vi "Get Strings from Ref (Ryan Porter's conflicted copy 2015-04-14).vi"(8 "error in (no error)":errorcluster, 9 "Label Prefix":string, 10 "GObj Refnum in":refnum<vi>, 11 "ArrayConstant in":refnum<class "ArrayControl.lvclass">) -> (0 "error out":errorcluster, 1 "Valid?":bool, 2 "GObj Refnum out":refnum<vi>, 3 "ArrayConstant out":refnum<class "ArrayControl.lvclass">, 4 "GObj Name":string)   [LabVIEW 2013, in "SET Project Data.lvlib" / "ArrayControl.lvclass"]
uses:
  ArrayControl.lvclass
  GObject/GObject.lvclass
  SET Project Data.lvlib
  Control/Control.lvclass
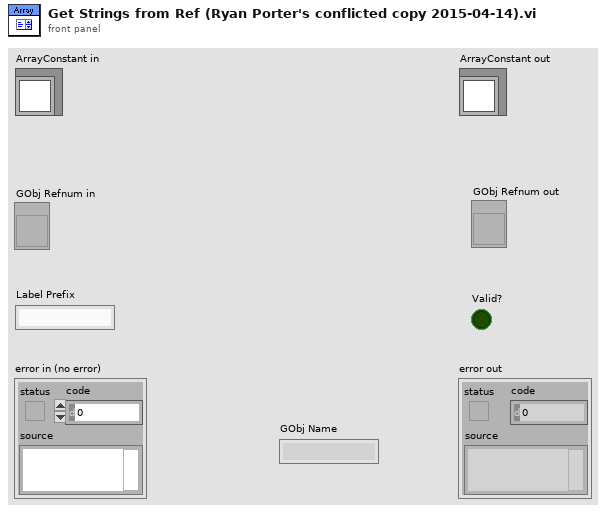
[diagram p1: front panel]
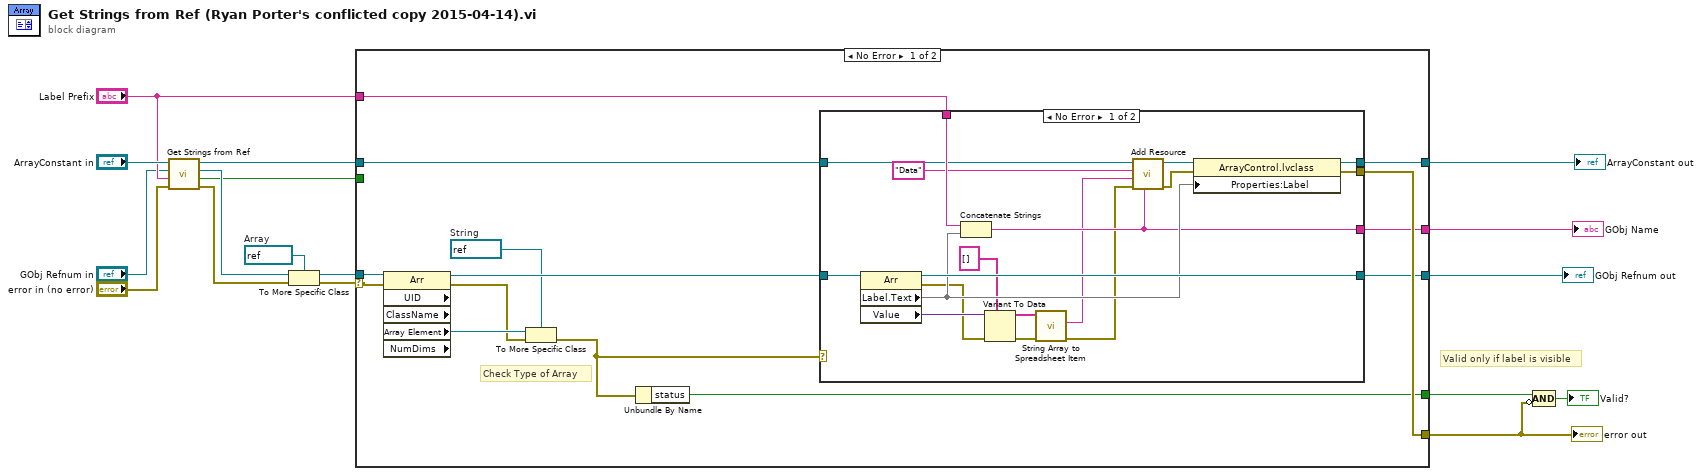
[diagram p0: block diagram]
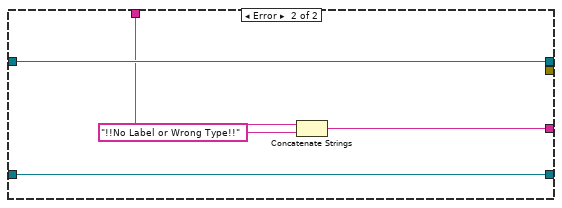
[diagram p2: hidden frame]
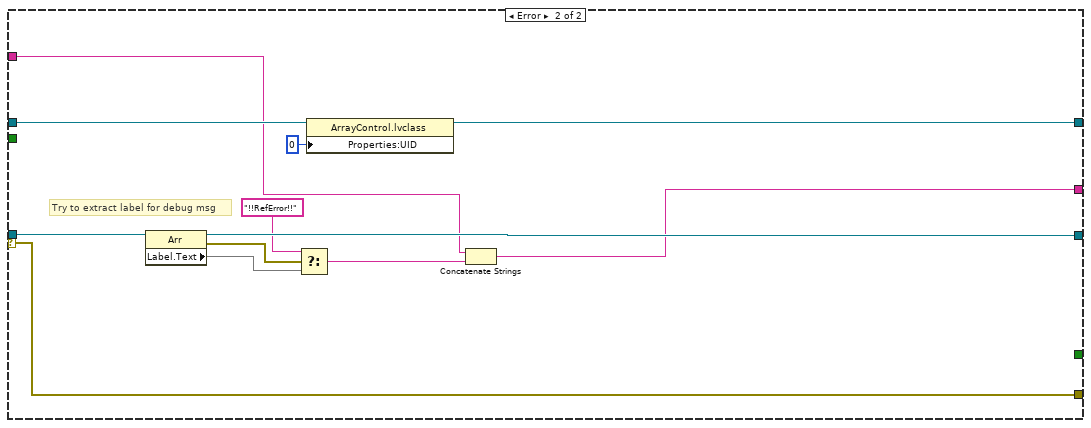
[diagram p3: hidden frame]
diagram:
  w9 = refnum<vi> refnum  # Array
  # "Valid only if label is visible"
  n1 = call-parent "Get Strings from Ref.vi"("error in (no error)"="error in (no error)", "Label Prefix"="Label Prefix", "GObj Refnum in"="GObj Refnum in", "Control in"="ArrayConstant in") -> ("error out"=w5:errorcluster, "Valid?"=w1:bool, "GObj Refnum out"=w2:refnum<vi>, "Control out"=w7:refnum<class "ArrayControl.lvclass">)  [unwired: 3 in, 1 out]
  n2 = To More Specific Class(target class=w9, reference=w2, error in=w5) -> (specific class reference=w16:refnum<vi>, error out=w15:errorcluster)
  n3 = case shown="No Error" w15 {
    selector: w15 -> [w28 w65]
    tunnel: w16 -> [w31 w61]
    tunnel: [w26 w60] -> w12
    tunnel: [w27 w65] -> w10
    tunnel: w7 -> [w18 w64]
    tunnel: [w30 w62] -> w14
    tunnel: "Label Prefix" -> [w25 w55]
    tunnel: [w19 _] -> w17
    tunnel: [w24 w59] -> w13
    tunnel: w1 -> [_ _]
    frame No Error {
      w21 = refnum<vi> refnum  # String
      # "Check Type of Array"
      n4 = property class="Arr" props=["UID", "ClassName", "Array Element", "NumDims"](reference=w31, error in=w28) -> (reference out=w29:refnum<vi>, error out=w22:errorcluster, "Array Element"=w23:refnum<vi>)  [unwired: 3 out]
      n5 = To More Specific Class(target class=w21, reference=w23, error in=w22) -> (error out=w20:errorcluster)  [unwired: 1 out]
      n6 = Unbundle By Name(w20) -> ("status"=w19:bool)
      n7 = case shown="No Error" w20 {
        tunnel: w18 -> [w43 w53]
        tunnel: [w48 w53] -> w30
        tunnel: w29 -> [w47 w52]
        tunnel: [w46 _] -> w27
        tunnel: [w45 w52] -> w26
        tunnel: w25 -> [w44 w51]
        tunnel: [w38 w49] -> w24
        frame No Error {
          n8 = property class="Arr"(reference=w47) -> (reference out=w45:refnum<vi>, error out=w33:errorcluster, "Label.Text"=w39, "Value"=w37:variant)  [unwired: 1 in]
          n9 = Concatenate Strings(w44, w39) -> (w38:string)
          n10 = Variant To Data(error in=w33, type=string[] [], Variant=w37) -> (data=w35:string[], error out=w32:errorcluster)
          n11 = call "String Array to Spreadsheet Item.vi"("Strings [] (ASCII)"=w35) -> ("Spreadsheet Item (ASCII)"=w34:string)  [unwired: 10 in]
          n12 = call "Add Resource.vi"("TagPrefix"=w38, "error in (no error)"=w32, "ItemText"=w34, "ItemName"="Data" ("name"), "GObject in"=w43) -> ("error out"=w40:errorcluster, "GObject out"=w42:refnum<class "ArrayControl.lvclass">)  [unwired: 5 in]
          n13 = property class="ArrayControl.lvclass"(reference=w42, error in=w40, "Properties:Label"=w39) -> (reference out=w48:refnum<class "ArrayControl.lvclass">, error out=w46:errorcluster)
        }
        frame Error {
          n14 = Concatenate Strings(w51, "!!No Label or Wrong Type!!") -> (w49:string)
        }
      }
    }
    frame Error {
      # "Try to extract label for debug msg"
      n15 = property class="Arr"(reference=w61) -> (reference out=w60:refnum<vi>, error out=w58:errorcluster, "Label.Text"=w56)  [unwired: 1 in]
      n16 = Select(t="!!RefError!!" ("Label.Text"), s=w58, f=w56) -> (s? t:f=w54:string)
      n17 = property class="ArrayControl.lvclass"(reference=w64, "Properties:UID"=0 ("UID")) -> (reference out=w62:refnum<class "ArrayControl.lvclass">)  [unwired: 1 in, 1 out]
      n18 = Concatenate Strings(w55, w54) -> (w59:string)
    }
  }
  "error out" <- w10
  "ArrayConstant out" <- w14
  "GObj Refnum out" <- w12
  "GObj Name" <- w13
  n19 = Compound Arithmetic op=AND(w17, invert w10) -> (→"Valid?":bool)
